vi "Wire Case selector from error wire.vi"   [LabVIEW 2012]
uses:
  Scripting Tools.lvlib
panel:
  # "Attempting to wire selected case structure(s) up to\nerror cluster wire"
types:
  T1 = enum16{"Case Structure", "Stacked Sequence", "Event Structure", "Diagram Disable", "Conditional Disable", "While Loop", "For Loop"}
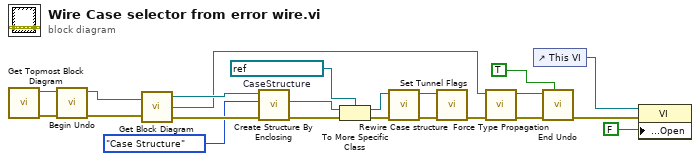
[diagram p0: block diagram]
diagram:
  w14 = refnum<vi> refnum  # CaseStructure
  n1 = call "Get Topmost Block Diagram.vi"() -> ("error out"=w11:errorcluster, "Vi refence for top most block diagram"=w10:refnum<vi>)  [unwired: 1 in, 9 out]
  n2 = call "Begin Undo.vi"("error in (no error)"=w11, "Vi Ref"=w10) -> ("error out"=w8:errorcluster, "Vi Ref Out"=w9:refnum<vi>)  [unwired: 1 in, 7 out]
  n3 = call "Get Block Diagram.vi"("vi refnum in"=w9, "error in (no error)"=w8) -> ("Diagram"=w19:refnum<vi>, "vi refnum out"=w4:refnum<vi>, "error out"=w20:errorcluster)
  n4 = call "Create Structure By Enclosing.vi"("error in (no error)"=w20, "Structure Type"=T1."Case Structure", "Diagram In"=w19) -> ("error out"=w17:errorcluster, "Structure Out"=w15:refnum<vi>)  [unwired: 1 in, 6 out]
  n5 = To More Specific Class(target class=w14, reference=w15, error in=w17) -> (specific class reference=w13:refnum<vi>, error out=w16:errorcluster)
  n6 = call "Rewire Case structure.vi"("error in (no error)"=w16, "CaseSel Refnum"=w13) -> ("error out"=w12:errorcluster, "CaseSel Refnum Out"=w5:refnum<vi>)  [unwired: 2 in, 6 out]
  n7 = call "Set Tunnel Flags.vi"("error in (no error)"=w12, "Struct Refnum"=w5) -> ("error out"=w1:errorcluster)  [unwired: 9 out]
  n8 = call "Force Type Propagation.vi"("error in (no error)"=w1, "reference"=w4) -> ("error out"=w3:errorcluster, "reference out"=w2:refnum<vi>)  [unwired: 1 in, 7 out]
  n9 = control-ref of="This VI"() -> (w21:refnum<vi>)
  n10 = call "End Undo.vi"("Successful Operation ?"=TRUE, "error in (no error)"=w3, "Vi Ref"=w2) -> ("error out"=w7:errorcluster)  [unwired: 8 out]
  n11 = property class="VI"(reference=w21, error in=w7, "Front Panel.Open"=FALSE ("Front Panel Window:Open")) -> ()  [unwired: 2 out]
